vi "Test-Meas HV Voltage.vi"(7 "Publishable ID":string, 8 "error in (no error)":errorcluster, 10 "Pins":string[](array[string])=["VDD"], 11 "Semiconductor Module Context":T1) -> (0 "error out":errorcluster)   [LabVIEW 2013]
uses:
  <vilib>/NI_TestStand_SemiconductorModule/NI_TestStand_Semiconductor_Module.lvlibp/PinMap/General/SemiconductorModuleContext.ctl
  <instrlib>/niDCPower/nidcpower.llb/niDCPower Measurement Type.ctl
  <vilib>/NI_TestStand_SemiconductorModule/NI_TestStand_Semiconductor_Module.lvlibp/PinMap/DC Power/PinsToNIDCPowerSessions.vi
  <vilib>/NI_TestStand_SemiconductorModule/NI_TestStand_Semiconductor_Module.lvlibp/PinMap/General/Publish/PublishDataDouble2D.vi
  <vilib>/NI_TestStand_SemiconductorModule/NI_TestStand_Semiconductor_Module.lvlibp
panel:
  out "Measurement":dbl[][](array[numeric])
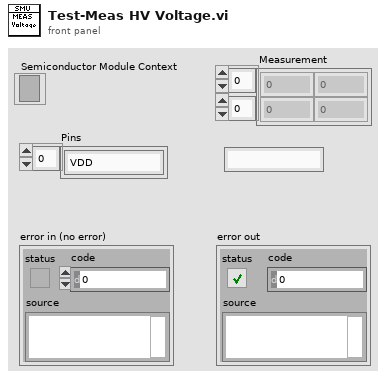
[diagram p1: front panel]
types:
  T1 = typedef "NI_TestStand_Semiconductor_Module.lvlibp/SemiconductorModuleContext.ctl" = refnum<k7>
  T2 = typedef "niDCPower Measurement Type.ctl" = i32
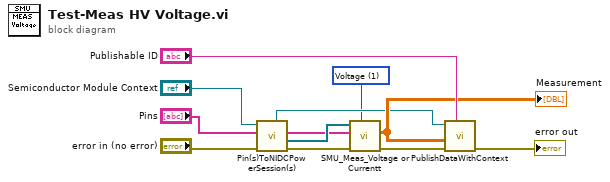
[diagram p0: block diagram]
diagram:
  w1 = T2 1 items=["Current", "Voltage"] ("measurement type")
  n1 = call-poly <vilib>:"Pin(s)ToNIDCPowerSession(s).vi"("error in (no error)"="error in (no error)", "Pins"="Pins", "Semiconductor Module Context"="Semiconductor Module Context") -> ("error out"=w9:errorcluster, "Instrument Sessions"=w8:refnum<k15>[], "Channel Lists"=w2:string[], "Pin Query Context"=w4:refnum<class "MultiplePinMultipleSessionQueryContext.lvclass">)  [unwired: 4 in, 1 out]
  n2 = call "SMU_Meas_Voltage or Currentt.vi"("measurement type"=w1, "error in (no error)"=w9, "Channel Lists"=w2, "DCPower Sessions In"=w8) -> ("error out"=w7:errorcluster, "Measurement"=w5:dbl[][])  [unwired: 5 in, 1 out]
  "Measurement" <- w5
  n3 = call-poly <vilib>:"PublishDataWithContext.vi"("Published Data Id"="Publishable ID", "error in (no error)"=w7, "Data In"=w5, "Pin Query Context"=w4) -> ("error out"=→"error out":errorcluster)  [unwired: 6 in, 1 out]
